vi "FTW-JSON-Core-LibraryError.vi"(0 "error in":errorcluster, 7 "Error Structure":u8[](array[numeric]) format="%02x") -> (4 "error out":errorcluster)   [LabVIEW 2013]
panel:
  # "Inputs"
  # "Outputs"
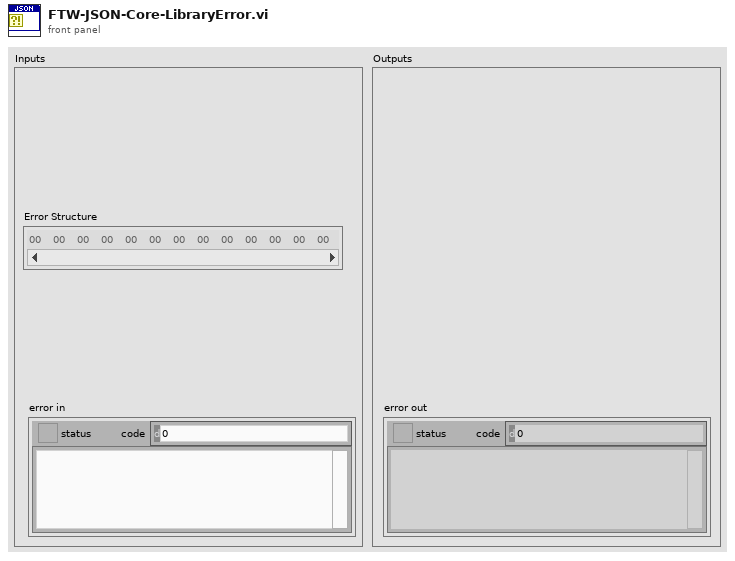
[diagram p1: front panel]
types:
  T1 = enum16{"big-endian, network order", "native, host order", "little-endian"}
  T2 = cluster{"Line Number":i32, "Column":i32, "Position":i32}
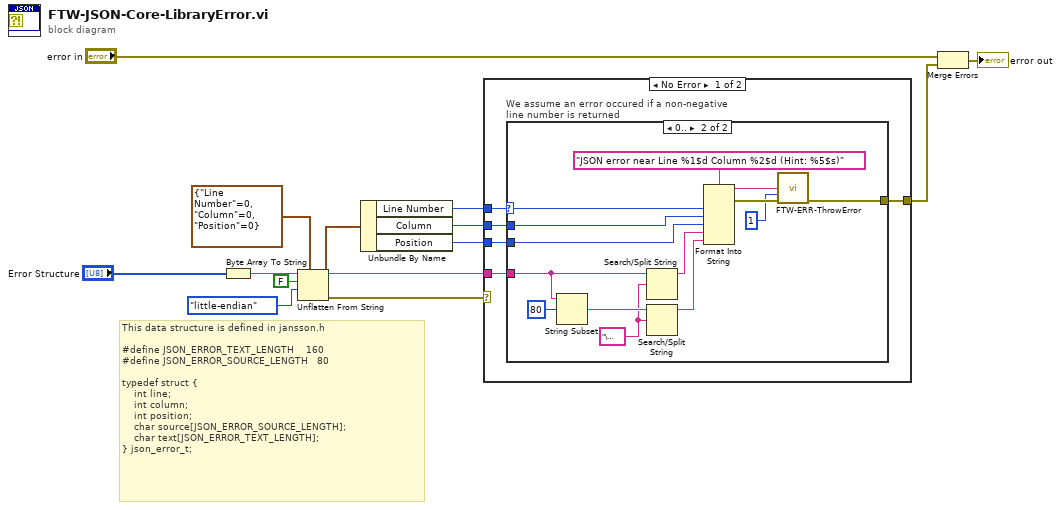
[diagram p0: block diagram]
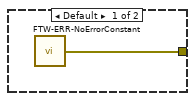
[diagram p2: hidden frame]
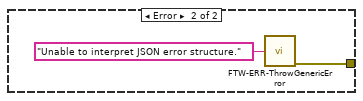
[diagram p3: hidden frame]
diagram:
  # "This data structure is defined in jansson.h\n\n#define JSON_ERROR_TEXT_LENGTH    160\n#define JSON_ERROR_SOURCE_LENGTH   80\n\ntypedef struct {\n    int line;\n    int column;\n    int position;\n    char source[JSON_ERROR_SOURCE_LENGTH];\n    char text[JSON_ERROR_TEXT_LENGTH];\n} json_error_t;"
  n1 = Byte Array To String(unsigned byte array="Error Structure") -> (string=w12:string)
  n2 = Unflatten From String(type=T2 {"Line Number"=0, "Column"=0, "Position"=0} ("error"), binary string=w12, data includes array or string size? (T)=FALSE, byte order (0:big-endian, network order)=T1."little-endian") -> (rest of the binary string=w6:string, value=w9:T2, error out=w4:errorcluster)  [unwired: 1 in]
  n3 = Unbundle By Name(w9) -> ("Line Number"=w5:i32, "Column"=w8:i32, "Position"=w7:i32)
  n4 = case shown="No Error" w4 {
    tunnel: w8 -> [w19 _]
    tunnel: w7 -> [w18 _]
    tunnel: w6 -> [w17 _]
    tunnel: w5 -> [w16 _]
    tunnel: [w15 w36] -> w3
    frame No Error {
      n5 = case "We assume an error occured if a non-negative line number is returned" shown="0.." w16 {
        selector: w16 -> [_ w22]
        tunnel: w19 -> [_ w32]
        tunnel: w18 -> [_ w31]
        tunnel: w17 -> [_ w28]
        tunnel: [w20 w21] -> w15
        frame Default {
          n6 = call "FTW-ERR-NoErrorConstant.vi"() -> ("no error"=w20:errorcluster)
        }
        frame 0.. {
          w27 = "\u0000" ("search string/char (-)")
          n7 = String Subset(string=w28, offset (0)=80) -> (substring=w29:string)  [unwired: 1 in]
          n8 = Search/Split String(string=w28, search string/char (-)=w27) -> (substring before match=w26:string)  [unwired: 1 in, 2 out]
          n9 = Search/Split String(string=w29, search string/char (-)=w27) -> (substring before match=w25:string)  [unwired: 1 in, 2 out]
          n10 = Format Into String(format string="JSON error near Line %1$d Column %2$d (Hint: %5$s)", w22, w32, w31, w26, w25) -> (resulting string=w33:string, error out=w24:errorcluster)  [unwired: 2 in]
          n11 = call "FTW-ERR-ThrowError.vi"("Error Message"=w33, "Error Code"=1, "error in"=w24) -> ("error out"=w21:errorcluster)  [unwired: 12 in]
        }
      }
    }
    frame Error {
      n12 = call "FTW-ERR-ThrowGenericError.vi"("Error Message"="Unable to interpret JSON error structure.") -> ("error out"=w36:errorcluster)  [unwired: 14 in]
    }
  }
  n13 = Merge Errors("error in", w3) -> (→"error out":errorcluster)
